vi "Config Format.vi"(0 "VISA resource name":refnum<visa-resource-name>, 1 "Notation (floating)":u16(ring) items=["Floating", "Scientific", "Engineering"], 2 "Lasbelling (on)":enum16{"off", "on"}(ring)=enum."on", 3 "Field Width (fixed)":u16(ring) items=["Fixed", "Variable"], 4 "Line End (CR-LF)":u16(ring) items=["CR_LF", "Semicolon"], 5 "Quotes (off)":enum16{"off", "on"}(ring), 7 "error in":errorcluster) -> (20 "VISA resource name out":refnum<visa-resource-name>, 27 "error out":errorcluster)   [LabVIEW 2019, in "Andeen-Hagerling 2700(400 firmware).lvlib"]
doc: "Controls the format and numeric notation of results which are sent to serial or GPIB ports. Front panel results are not affected."
uses:
  Andeen-Hagerling 2700(400 firmware).lvlib
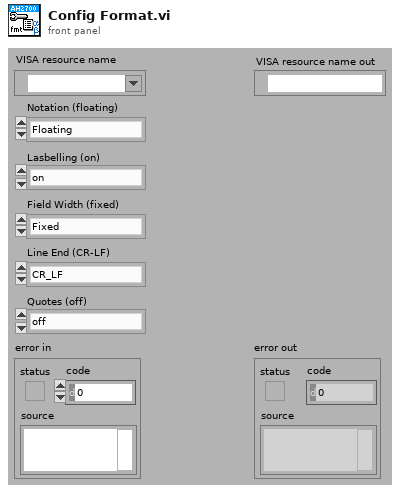
[diagram p1: front panel]
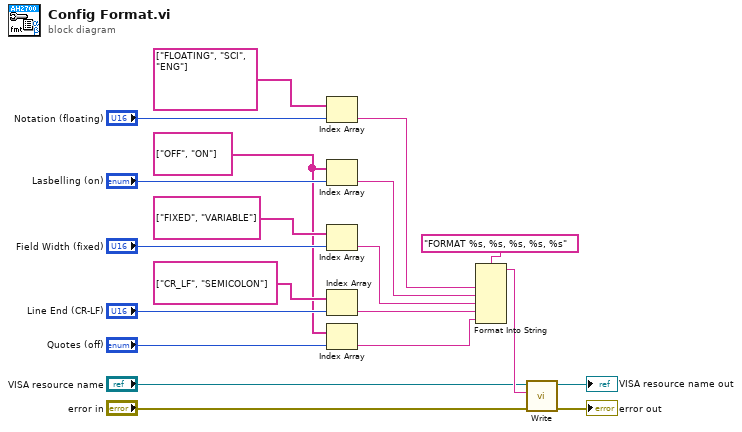
[diagram p0: block diagram]
diagram:
  w3 = string[] ["OFF", "ON"]
  n1 = Index Array(array=string[] ["FLOATING", "SCI", "ENG"], index="Notation (floating)") -> (element=w11:string)
  n2 = Index Array(array=w3, index="Lasbelling (on)") -> (element=w10:string)
  n3 = Index Array(array=string[] ["FIXED", "VARIABLE"], index="Field Width (fixed)") -> (element=w7:string)
  n4 = Index Array(array=string[] ["CR_LF", "SEMICOLON"], index="Line End (CR-LF)") -> (element=w5:string)
  n5 = Index Array(array=w3, index="Quotes (off)") -> (element=w1:string)
  n6 = Format Into String(format string="FORMAT %s, %s, %s, %s, %s", w11, w10, w7, w5, w1) -> (resulting string=w20:string)  [unwired: 2 in, 1 out]
  n7 = call "Write.vi"("error in"="error in", "command"=w20, "VISA resource name"="VISA resource name") -> ("error out"=→"error out":errorcluster, "VISA resource name out"=→"VISA resource name out":refnum<visa-resource-name>)  [unwired: 7 in]
